vi "Handle Command.vi"(5 "Preceding Items":refnum<class "Item.lvclass">[](array[class]), 7 "Command":string, 8 "error in (no error)":errorcluster, 9 "Active Build Configuration":string, 10 "Selected Items":string[][](array[string]), 11 "Caraya Item in":refnum<class "Caraya Item.lvclass">) -> (0 "error out":errorcluster, 1 "Steps to Build":refnum<class "Build Step.lvclass">[](array[class]), 2 "LV Documents to Open":path[](array[path]), 3 "Caraya Item out":refnum<class "Caraya Item.lvclass">)   [LabVIEW 2019, in "Caraya Library.lvlib" / "Caraya Item.lvclass"]
uses:
  Caraya Item.lvclass
  libs/Solution.lvlibp/Solution/Item/Item.lvclass
  libs/Solution.lvlibp/Solution/Build Item/Build Step.lvclass
  Caraya Item.lvclass/Caraya Item.ctl
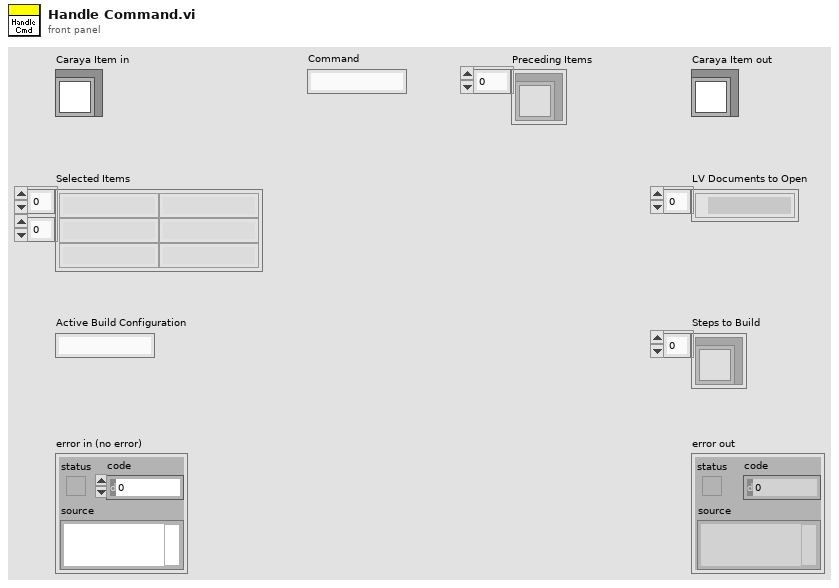
[diagram p1: front panel]
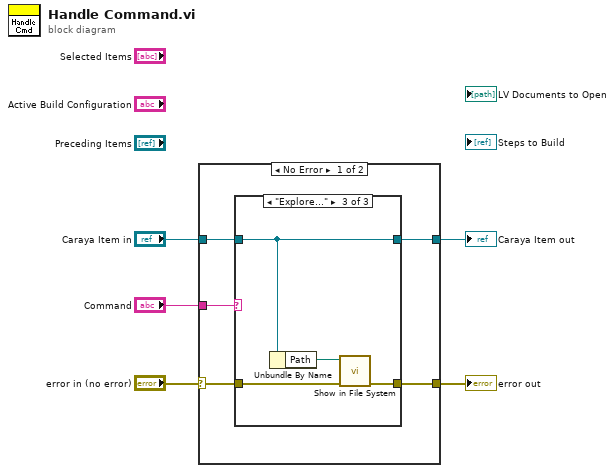
[diagram p0: block diagram]
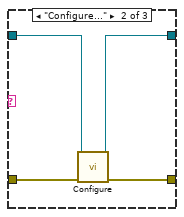
[diagram p3: hidden frame]
diagram:
  n1 = case shown="No Error" "error in (no error)" {
    selector: "error in (no error)" -> [w10 w21]
    tunnel: [w9 w21] -> w4
    tunnel: "Caraya Item in" -> [w8 w22]
    tunnel: [w7 w22] -> w2
    tunnel: "Command" -> [w6 _]
    frame No Error {
      n2 = case shown="\"Explore...\"" w6 {
        tunnel: w10 -> [w11 w16 w20]
        tunnel: [w11 w15 w19] -> w9
        tunnel: w8 -> [w12 w14 w18]
        tunnel: [w12 w13 w18] -> w7
        frame Default {
        }
        frame "Configure..." {
          n3 = call "Configure.vi"("error in (no error)"=w16, "Caraya Item in"=w14) -> ("error out"=w15:errorcluster, "Caraya Item out"=w13:refnum<class "Caraya Item.lvclass">)  [unwired: 8 in]
        }
        frame "Explore..." {
          n4 = Unbundle By Name(w18) -> ("Path"=w17:path)
          n5 = call <vilib>:"Show in File System.vi"("error in (no error)"=w20, "file or directory path"=w17) -> ("error out"=w19:errorcluster)  [unwired: 9 in]
        }
      }
    }
    frame Error {
    }
  }
  "error out" <- w4
  "Caraya Item out" <- w2
